vi "Read and Unflatten.vi"(8 "error in (no error)":errorcluster, 9 "Timeout (ms)":i32, 10 "Data in":T2[](array[typedef]), 11 "CIF_NIChn_FIFO_DAQ in":refnum<class "CIF_NIChn_FIFO_DAQ.lvclass">) -> (0 "error out":errorcluster, 1 "Timed out?":bool, 2 "Data out":T2[](array[typedef]), 3 "CIF_NIChn_FIFO_DAQ out":refnum<class "CIF_NIChn_FIFO_DAQ.lvclass">, 4 "Header out":T1)   [LabVIEW 2021, in "CIF_NIChn_FIFO_DAQ.lvclass"]
uses:
  CIF_NIChn_FIFO_DAQ.lvclass
  D:/dev/Packages/Channel_Manager/src/CIF_NIChn/NIChn/CIF_NIChn.lvclass
  D:/dev/Packages/Channel_Manager/src/CIFChannels/CIFChannels.lvclass
  ChannelCommon/typedef/Datatype Waveform.ctl
  ChannelCommon/typedef/FIFO Header.ctl
  NIChn/CIF_NIChn.lvclass/CIF_NIChn.ctl
  CIFChannels/CIFChannels.lvclass/CIFChannels.ctl
  <vilib>/CIF Foundation/CIF Utilities/Statistics/I64/Stats_I64_CIF_U.lvclass/Stats_I64_CIF_U.ctl
  8d434fcd-ba02-44c6-a1d2-d54d1c5f4ff9.vi
  c632fbd8-b242-46ac-b145-31e81b296fef.vi
  ChannelCommon/Utilities/Add Error.vi
  <vilib>/CIF Foundation/CIF Channels/CIFChannels/Top Level/Read U8 Array.vi/4bc1c15b-36ab-481f-b8dd-c64075ce723a.vi
  <vilib>/CIF Foundation/CIF Channels/CIFChannels/Top Level/Read U8 Array.vi/d83cb72b-7713-41fc-a3d1-682de79cf574.vi
  <vilib>/CIF Foundation/CIF Channels/CIFChannels/SubVIs/Get dll Path.vi
  <vilib>/CIF Foundation/CIF Channels/CIFChannels/SubVIs/Get Requested Size.vi
  <vilib>/CIF Foundation/CIF Channels/CIFChannels/Top Level/Advanced/Read U8 FIFO as Dbl Array.vi/4bc1c15b-36ab-481f-b8dd-c64075ce723a.vi
  <vilib>/CIF Foundation/CIF Channels/CIFChannels/Top Level/Advanced/Read U8 FIFO as Dbl Array.vi/d83cb72b-7713-41fc-a3d1-682de79cf574.vi
  <vilib>/CIF Foundation/CIF Utilities/Statistics/I64/X1 minus X0.vi
  <vilib>/CIF Foundation/CIF Utilities/Time/System Time/Get System Time.vi
  <vilib>/CIF Foundation/CIF Utilities/Errors/Append Error Location.vi
  <vilib>/CIF Foundation/CIF Utilities/Statistics/I64/X1 minus X0.vi/dfabcf33-0dbc-4041-80a5-3dc0c86d2989.vi
  <vilib>/CIF Foundation/CIF Utilities/Time/System Time/LabVIEW Time to TAI Time.vi
  <vilib>/CIF Foundation/CIF Utilities/Statistics/I64/X1 minus X0.vi/dfabcf33-0dbc-4041-80a5-3dc0c86d2989.vi/9eb60a9a-770f-4d2d-8b3f-8465c267ecc9.vi
  NIChn/CIF_NIChn.lvclass
  ChannelCommon/ChannelCommon.lvlib
  <vilib>/CIF Foundation/CIF Utilities/DataTypes/DataTypes_CIF_U.lvlib
  <vilib>/CIF Foundation/CIF Channels/CIFChannels/CIFChannelCore.lvlib
  CIFChannels/CIFChannels.lvclass
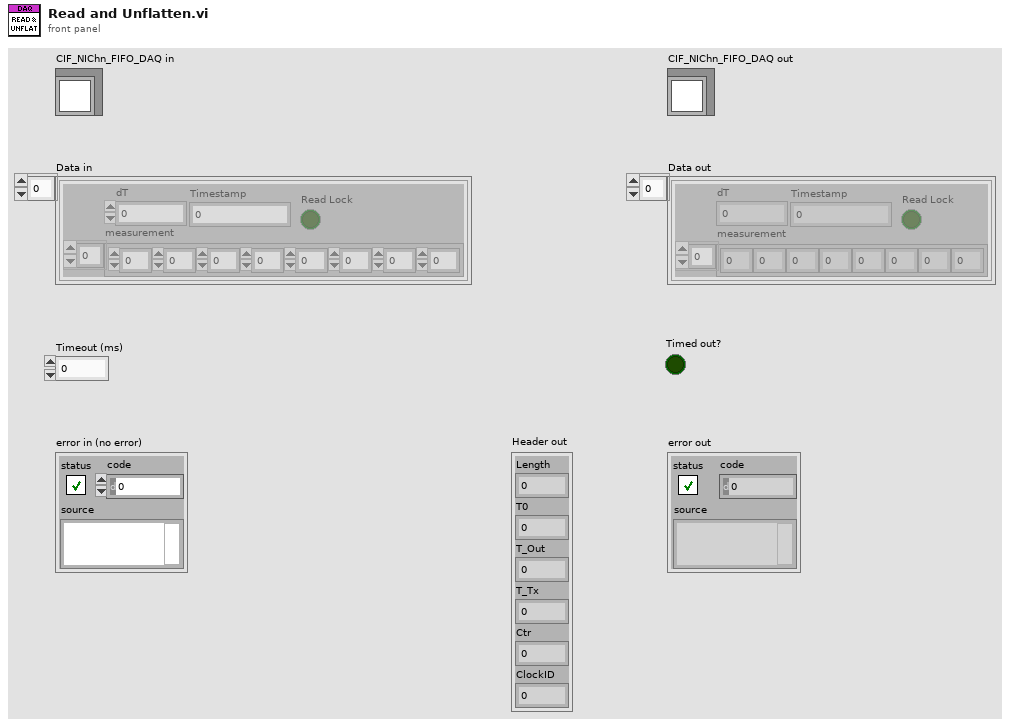
[diagram p1: front panel]
types:
  T1 = typedef "ChannelCommon.lvlib/FIFO Header.ctl" = cluster{"Length":u64, "T0":i64, "T_Out":i64, "T_Tx":i64, "Ctr":u64, "ClockID":u8}
  T2 = typedef "ChannelCommon.lvlib/Datatype Waveform.ctl" = cluster{"measurement":dbl[], "dT":dbl, "Timestamp":i64, "Read Lock":bool}
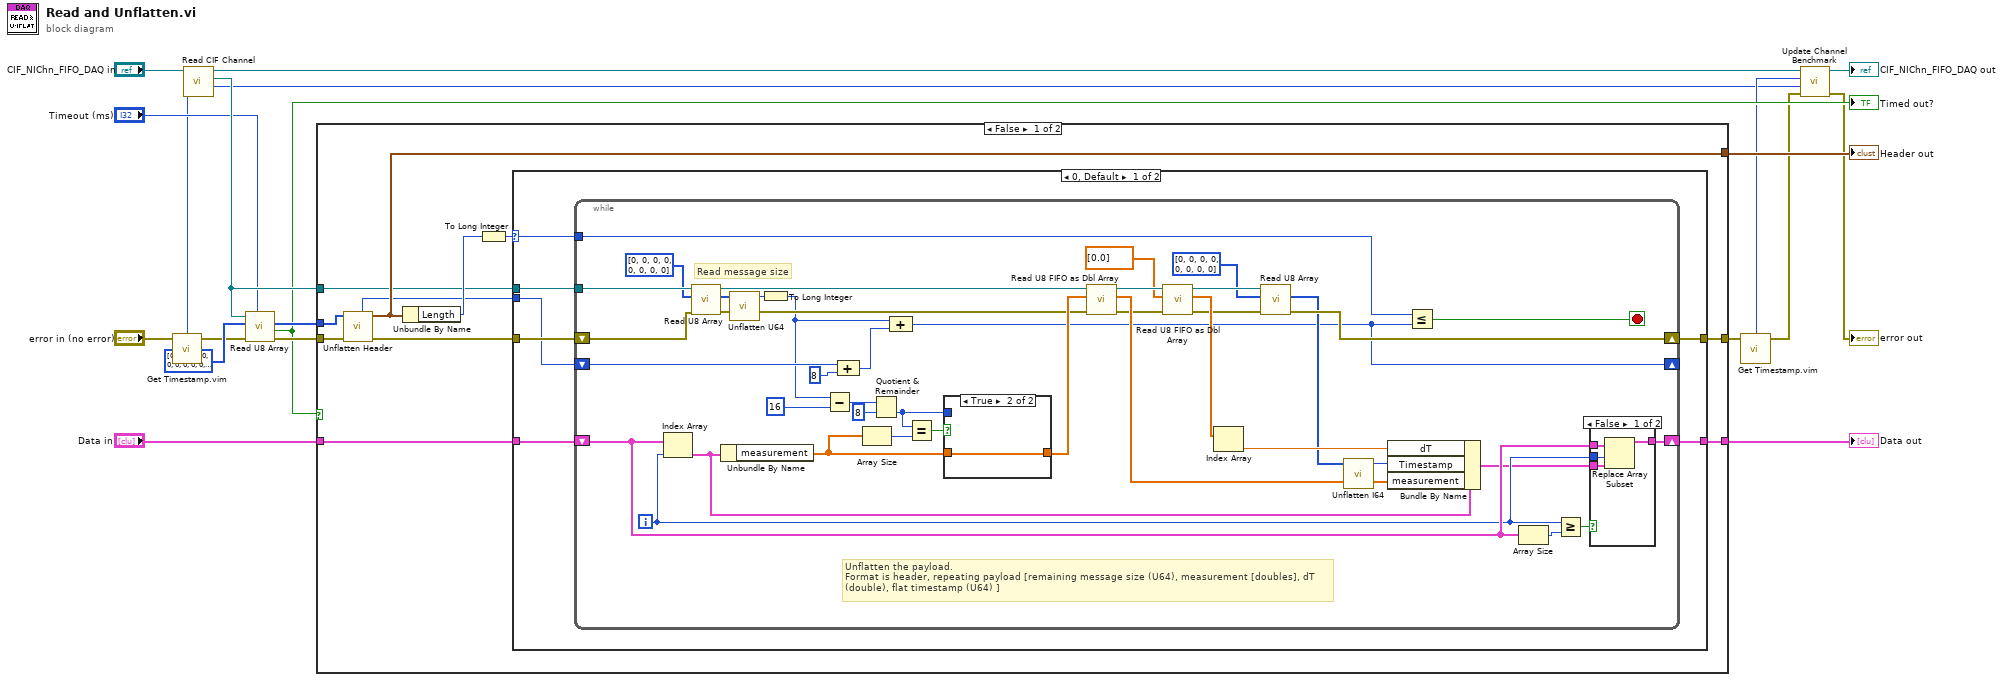
[diagram p0: block diagram]
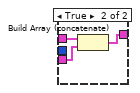
[diagram p2: hidden frame]
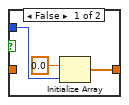
[diagram p3: hidden frame]
diagram:
  n1 = call "Get Timestamp.vim"("Anything in"="error in (no error)") -> ("Time (ns)"=w1:i64, "Anything out"=w2:errorcluster)  [unwired: 2 in]
  n2 = call "Read CIF Channel.vi"("CIFTag in"="CIF_NIChn_FIFO_DAQ in") -> ("CIF Channel"=w13:refnum<k21>, "CIFTag out"=w9:refnum<class "CIF_NIChn_FIFO_DAQ.lvclass">)  [unwired: 8 in, 1 out]
  n3 = call <vilib>:"Read U8 Array.vi"("Timeout (ms)"="Timeout (ms)", "error in"=w2, "U8 Array in"=u8[] [0, 0, 0, 0, 0, 0, 0, 0, 0, 0, 0, 0, 0, 0, 0, 0, 0, 0, 0, 0, 0, 0, 0, 0, 0, 0, 0, 0, 0, 0, 0, 0, 0, 0, 0, 0, 0, 0, 0, 0, 0, 0, 0, 0, 0, 0, 0, 0], "CIF Channel in"=w13) -> ("error out"=w14:errorcluster, "Timed out?"=w12:bool, "U8 Array out"=w15:u8[])  [unwired: 4 in, 1 out]
  "Timed out?" <- w12
  n4 = case shown="False" w12 {
    tunnel: [w30 w92] -> w19
    tunnel: "Data in" -> [w29 w92]
    tunnel: [w26 _] -> w17
    tunnel: w15 -> [w20 _]
    tunnel: w14 -> [w24 w93]
    tunnel: w13 -> [w23 _]
    tunnel: [w22 w93] -> w6
    frame False {
      n5 = call "Unflatten Header.vi"("error in (no error)"=w24, "Flattened Data in"=w20) -> ("error out"=w28:errorcluster, "Header out"=w26:T1, "offset out"=w21:i32)  [unwired: 7 in]
      n6 = Unbundle By Name(w26) -> ("Length"=w27:u64)
      n7 = To Long Integer(number=w27) -> (32bit integer=w25:i32)
      n8 = case shown="0, Default" w25 {
        selector: w25 -> [w33 _]
        tunnel: [w37 w90] -> w30
        tunnel: w29 -> [w36 w90]
        tunnel: [w35 w91] -> w22
        tunnel: w28 -> [w34 w91]
        tunnel: w23 -> [w32 _]
        tunnel: w21 -> [w31 _]
        frame 0, Default {
          n9 = while {
            shift-right: [w76] -> w35
            shift-left: w34 -> [w77]
            shift-right: [w38] -> _
            shift-left: w31 -> [w78]
            tunnel: w33 -> [w75]
            shift-right: [w73] -> w37
            shift-left: w36 -> [w43]
            tunnel: w32 -> [w72]
            i -> [w42]
            stop <- w74 stop-if-true
            # "Read message size"
            # "Unflatten the payload.\nFormat is header, repeating payload [remaining message size (U64), measurement [doubles], dT (double), flat timestamp (U64) ]"
            n10 = Index Array(array=w43, index=w42) -> (element=w71:T2)
            n11 = call <vilib>:"Read U8 Array.vi"("error in"=w77, "U8 Array in"=u8[] [0, 0, 0, 0, 0, 0, 0, 0], "CIF Channel in"=w72) -> ("error out"=w56:errorcluster, "U8 Array out"=w60:u8[], "CIF Channel out"=w58:refnum<k21>)  [unwired: 5 in, 1 out]
            n12 = Unbundle By Name(w71) -> ("measurement"=w62:dbl[])
            n13 = call <vilib>:"Unflatten U64.vi"("Flat Data"=w60) -> ("U64"=w59:u64)  [unwired: 4 in]
            n14 = To Long Integer(number=w59) -> (32bit integer=w44:i32)
            n15 = Subtract(x=w44, y=16) -> (x-y=w65:i32)
            n16 = Compound Arithmetic op=ADD(w78, 8 ("value")) -> (w68:i32)
            n17 = Array Size(array=w62) -> (size(s)=w67:i32)
            n18 = Quotient & Remainder(x=w65, y=8) -> (floor(x/y)=w64:i32)  [unwired: 1 out]
            n19 = Compound Arithmetic op=ADD(w44, w68) -> (w38:i32)
            n20 = Equal?(x=w64, y=w67) -> (x = y?=w66:bool)
            n21 = case shown="True" w66 {
              tunnel: w62 -> [_ w89]
              tunnel: [w86 w89] -> w57
              tunnel: w64 -> [w88 _]
              frame False {
                n22 = Initialize Array(0.0, w88) -> (w86:dbl[])
              }
              frame True {
              }
            }
            n23 = call <vilib>:"Read U8 FIFO as Dbl Array.vi"("error in"=w56, "DBL Array in"=w57, "CIF Channel in"=w58) -> ("error out"=w53:errorcluster, "DBL Array out"=w55:dbl[], "CIF Channel out"=w54:refnum<k21>)  [unwired: 5 in, 1 out]
            n24 = call <vilib>:"Read U8 FIFO as Dbl Array.vi"("error in"=w53, "DBL Array in"=dbl[] [0.0], "CIF Channel in"=w54) -> ("error out"=w45:errorcluster, "DBL Array out"=w51:dbl[], "CIF Channel out"=w49:refnum<k21>)  [unwired: 5 in, 1 out]
            n25 = Index Array(array=w51) -> (element=w50:dbl)  [unwired: 1 in]
            n26 = call <vilib>:"Read U8 Array.vi"("error in"=w45, "U8 Array in"=u8[] [0, 0, 0, 0, 0, 0, 0, 0], "CIF Channel in"=w49) -> ("error out"=w76:errorcluster, "U8 Array out"=w47:u8[])  [unwired: 5 in, 2 out]
            n27 = call <vilib>:"Unflatten I64.vi"("Flat Data"=w47) -> ("I64"=w46:i64)  [unwired: 4 in]
            n28 = Bundle By Name(cluster=w71, "dT"=w50, "Timestamp"=w46, "measurement"=w55) -> (w39:T2)
            n29 = Less Or Equal?(x=w75, y=w38) -> (x <= y?=w74:bool)
            n30 = Array Size(array=w43) -> (size(s)=w41:i32)
            n31 = Greater Or Equal?(x=w42, y=w41) -> (x >= y?=w40:bool)
            n32 = case shown="False" w40 {
              tunnel: [w82 w83] -> w73
              tunnel: w39 -> [w81 w84]
              tunnel: w43 -> [w80 w85]
              tunnel: w42 -> [w79 _]
              frame False {
                n33 = Replace Array Subset(array=w80, new element=w81, index=w79) -> (w82:T2[])
              }
              frame True {
                n34 = Build Array (concatenate)(w85, w84) -> (w83:T2[])
              }
            }
          }
        }
        frame 48 {
        }
      }
    }
    frame True {
    }
  }
  "Data out" <- w19
  "Header out" <- w17
  n35 = call "Get Timestamp.vim"("Anything in"=w6) -> ("Time (ns)"=w4:i64, "Anything out"=w5:errorcluster)  [unwired: 2 in]
  n36 = call "Update Channel Benchmark.vi"("error in (no error)"=w5, "X0"=w1, "X1"=w4, "CIFChannels in"=w9) -> ("error out"=→"error out":errorcluster, "CIFChannels out"=→"CIF_NIChn_FIFO_DAQ out":refnum<class "CIF_NIChn_FIFO_DAQ.lvclass">)  [unwired: 6 in]
